vi "SlaveAccelerometerSample6.vi"   [LabVIEW 2018]
uses:
  DataTypes/AccelerometerRecord.ctl
  <vilib>/rvi/Emulation/niFpgaGetClockAttributes.vi
  <vilib>/rvi/Emulation/niFpgaSctlEmulationGetInTimedLoop.vi
  <vilib>/rvi/Emulation/niFpgaEmulationReportErrorSimple.vi
  <vilib>/rvi/eio/common/nirviEmuTemplateMethod_errors.vi
  <vilib>/rvi/Emulation/niFpgaEmulationIsFPGAContextNoSignature.vi
  <vilib>/rvi/DataTransferAndStorage/Container/Common/niFpgaContainerGetUniqueNameForEmu.vi
  <vilib>/rvi/Memory/Memory_Emulation/niFpgaMemoryEmulationCacheClearOnFirstRun.vi
  <vilib>/rvi/Memory/Memory_Emulation/nirvimemoryEmulationManagerCache_MakeExclusive.vi
  <vilib>/rvi/Memory/Memory_Emulation/niFpgaMemoryEmulationValidateCache.vi
  <vilib>/rvi/Memory/Memory_Emulation/nirvimemoryEmulationManagerCache_InsertValue.vi
  <vilib>/Utility/error.llb/Clear Errors.vi
  <vilib>/rvi/Memory/Memory_Emulation/nirvimemoryEmulationManagerCache_ReleaseExclusive.vi
  <vilib>/rvi/Memory/Memory_Emulation/nirvimemoryEmulationManagerCache_GetValue.vi
  <vilib>/rvi/Memory/Memory_Emulation/nirvimemoryEmulationManagerCache_SetValue.vi
  <vilib>/rvi/Emulation/niFpgaProcessEmulError.vi
  <vilib>/rvi/errors/niFpgaSetErrorForExecOnDevCompSimple.vi
  <vilib>/rvi/eio/common/nirviEmuReportErrorAndStop.vi
  <vilib>/rvi/FIFO/Fifo_Resource/nirvififoEmulationSetSize.vi
  <vilib>/rvi/FIFO/Fifo_Resource/nirviFifoEmulationQueueMgr.vi
  <instcachedir>/0/nirviFifoEmulationQueueMgr_E5CAEC123FF24DC58D834DCA3CDAA9B5.lvgen/nirviFifoEmulationQueueMgr_E5CAEC123FF24DC58D834DCA3CDAA9B5_032.vi
  <vilib>/rvi/FIFO/Fifo_Resource/nirvififoEmulationDetermineInputValidOut.vi
  <vilib>/rvi/FIFO/Fifo_Resource/nirvififoEmulationCreateLock.vi
  <vilib>/rvi/FIFO/Fifo_Resource/nirvififoEmulationObtainLock.vi
  <vilib>/rvi/FIFO/Fifo_Resource/nirvififoEmulationReleaseLock.vi
  <vilib>/rvi/occurrence/nirviWaitOnOccurrenceBase.vi
  <vilib>/rvi/errors/nirviReportUnexpectedCaseInternalError.vi
  <vilib>/rvi/errors/nirviReportUnexpectedCaseInternalError (U32).vi
  <vilib>/rvi/Emulation/niFpgaCriticalErrorInLSC.vi
  <vilib>/eio/EIOMethodNode/EIOMethodNode.xnode
  <vilib>/rvi/DataTransferAndStorage/Container/XNode/niFpgaContainer.xnode
  <vilib>/rvi/DataTransferAndStorage/Register/Emulation/niFpgaRegisterEmulation.vi
  <vilib>/eio/EIONode/EIONode.xnode
  <vilib>/rvi/FIFO/Fifo_Resource/nirvififoEmulationWrite.vi
types:
  T1 = typedef "AccelerometerRecord.ctl" = cluster{"Timestamp":u64, "Accelerometers":sgl[]}
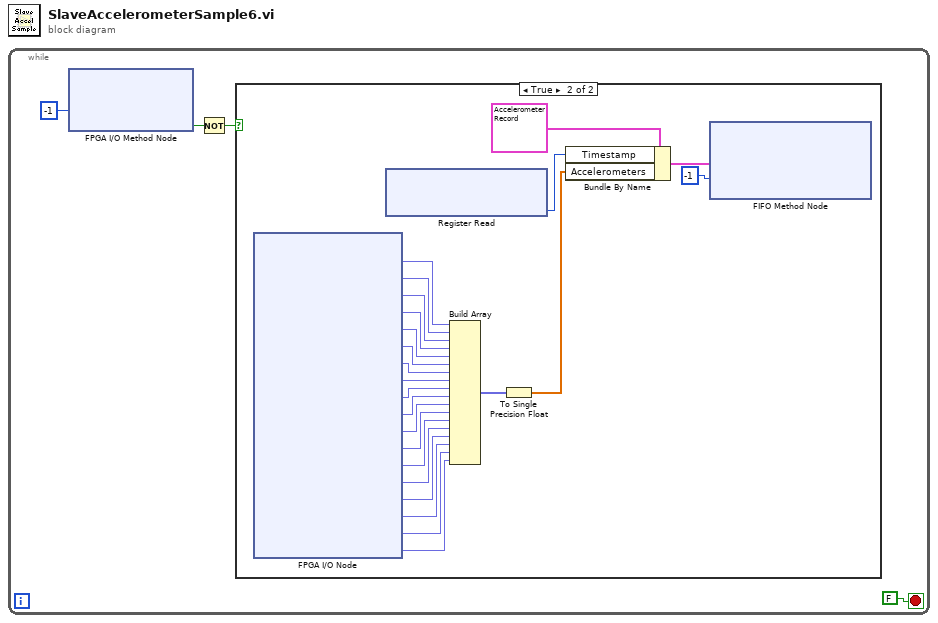
[diagram p0: block diagram]
diagram:
  n1 = while {
    stop <- FALSE stop-if-true
    n2 = xnode "FPGA I/O Method Node"("Timeout"=-1) -> ("Timed Out"=w2:bool)  [unwired: 1 in, 1 out]
    n3 = Not(x=w2) -> (.not. x?=w1:bool)
    n4 = case shown="True" w1 {
      frame False {
      }
      frame True {
        n5 = xnode "FPGA I/O Node"() -> ("Accelerometer1/AI0"=w27:fxp<+/-,24,7>, "Accelerometer1/AI1"=w26:fxp<+/-,24,7>, "Accelerometer1/AI2"=w25:fxp<+/-,24,7>, "Accelerometer2/AI0"=w24:fxp<+/-,24,7>, "Accelerometer2/AI1"=w23:fxp<+/-,24,7>, "Accelerometer2/AI2"=w22:fxp<+/-,24,7>, "Accelerometer3/AI0"=w21:fxp<+/-,24,7>, "Accelerometer3/AI1"=w20:fxp<+/-,24,7>, "Accelerometer3/AI2"=w19:fxp<+/-,24,7>, "Accelerometer4/AI0"=w18:fxp<+/-,24,7>, "Accelerometer4/AI1"=w17:fxp<+/-,24,7>, "Accelerometer4/AI2"=w16:fxp<+/-,24,7>, "Accelerometer5/AI0"=w15:fxp<+/-,24,7>, "Accelerometer5/AI1"=w14:fxp<+/-,24,7>, "Accelerometer5/AI2"=w13:fxp<+/-,24,7>, "Accelerometer6/AI0"=w12:fxp<+/-,24,7>, "Accelerometer6/AI1"=w11:fxp<+/-,24,7>, "Accelerometer6/AI2"=w10:fxp<+/-,24,7>)  [unwired: 18 in, 18 out]
        n6 = xnode ("Register Read")() -> ("Data"=w5:u64)  [unwired: 1 in, 1 out]
        n7 = Build Array(w27, w26, w25, w24, w23, w22, w21, w20, w19, w18, w17, w16, w15, w14, w13, w12, w11, w10) -> (w28:fxp<+/-,24,7>[])
        n8 = To Single Precision Float(number=w28) -> (single precision float=w6:sgl[])
        n9 = Bundle By Name(cluster=T1 {"Timestamp"=0, "Accelerometers"=[0.0, 0.0, 0.0, 0.0, 0.0, 0.0, 0.0, 0.0, 0.0, 0.0, 0.0, 0.0, 0.0, 0.0, 0.0, 0.0, 0.0, 0.0]} ("AccelerometerSample"), "Timestamp"=w5, "Accelerometers"=w6) -> (w7:T1)
        n10 = xnode ("FIFO Method Node")("Element"=w7, "Timeout"=-1) -> ()  [unwired: 1 in, 2 out]
      }
    }
  }
